vi "calculate virtual Z pos.vi"   [LabVIEW 2012]
uses:
  <vilib>/Analysis/coordinate.llb/Euler Rotation Order.ctl
  GFG/GFGnumericGet.vi
  <vilib>/Analysis/coordinate.llb/3D Cartesian Coordinate Rotation (Euler) (Scalar).vi
  <vilib>/Analysis/NI_AALPro.lvlib
  GFG/GFG library.lvlib
types:
  T1 = cluster{"Numeric":dbl, "Numeric":dbl, "Numeric":dbl}
  T2 = typedef "NI_AALPro.lvlib/Euler Rotation Order.ctl" = u16
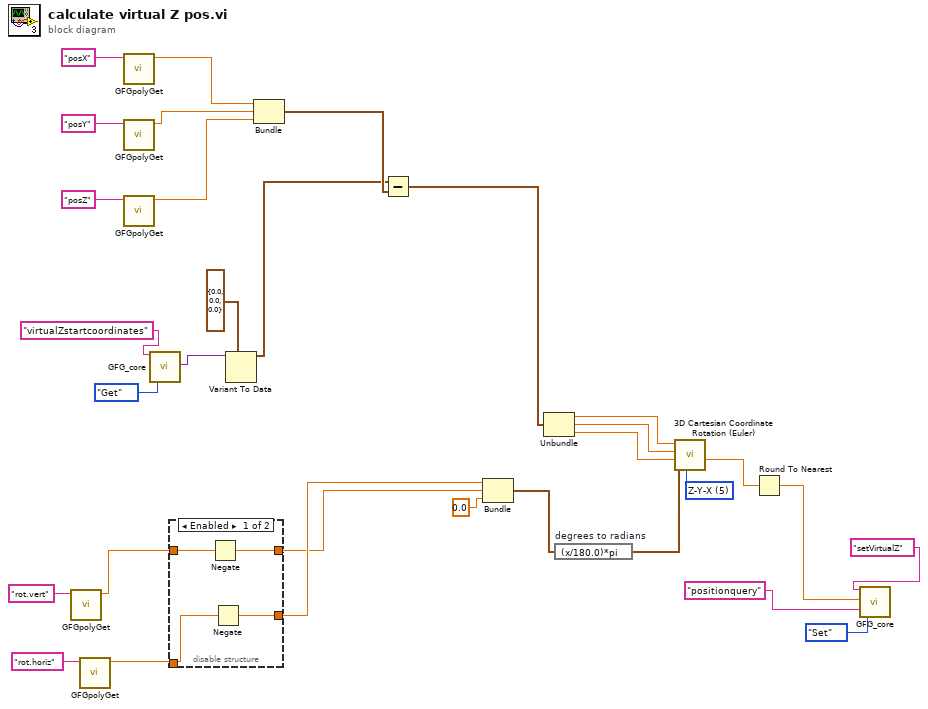
[diagram p0: block diagram]
diagram:
  w30 = T2 5 items=["X-Y-Z", "X-Z-Y", "Y-X-Z", "Y-Z-X", "Z-X-Y", "Z-Y-X", "X-Y-X", "X-Z-X", "Y-X-Y", "Y-Z-Y", "Z-X-Z", "Z-Y-Z"] ("rotation order")
  n1 = call-poly "GFGpolyGet.vi"("Variable Name in"="rot.vert") -> ("Numeric"=w14:dbl)  [unwired: 9 in, 1 out]
  n2 = call-poly "GFGpolyGet.vi"("Variable Name in"="rot.horiz") -> ("Numeric"=w15:dbl)  [unwired: 9 in, 1 out]
  n3 = call-poly "GFGpolyGet.vi"("Variable Name in"="posX") -> ("Numeric"=w22:dbl)  [unwired: 9 in, 1 out]
  n4 = call-poly "GFGpolyGet.vi"("Variable Name in"="posY") -> ("Numeric"=w21:dbl)  [unwired: 9 in, 1 out]
  n5 = call-poly "GFGpolyGet.vi"("Variable Name in"="posZ") -> ("Numeric"=w20:dbl)  [unwired: 9 in, 1 out]
  n6 = call "GFG_core.vi"("Variable Name in"="virtualZstartcoordinates", "Action"=enum16{"Init", "Set", "Get"}."Get") -> ("Variant Out"=w27:variant)  [unwired: 11 in, 6 out]
  n7 = disable-structure shown="Enabled" {
    disable-tunnel: w15 -> [w35 w36]
    disable-tunnel: w14 -> [w34 w37]
    disable-tunnel: [w33 w37] -> w7
    disable-tunnel: [w32 w36] -> w8
    frame Enabled {
      n8 = Negate(x=w34) -> (-x=w33:dbl)
      n9 = Negate(x=w35) -> (-x=w32:dbl)
    }
    frame Disabled {
    }
  }
  n10 = Variant To Data(type=T1 {"Numeric"=0.0, "Numeric"=0.0, "Numeric"=0.0} ("output cluster"), Variant=w27) -> (data=w18:T1)  [unwired: 1 in, 1 out]
  n11 = Bundle("Numeric"=w22, "Numeric"=w21, "Numeric"=w20) -> (w19:T1)  [unwired: 1 in]
  n12 = Subtract(x=w18, y=w19) -> (x-y=w13:T1)
  n13 = Bundle(w8, w7, "phi"=0.0) -> (w5:cluster{dbl, dbl, "phi":dbl})  [unwired: 1 in]
  n14 = Unbundle(w13) -> ("Numeric"=w12:dbl, "Numeric"=w11:dbl, "Numeric"=w10:dbl)
  n15 = expression code="(x/180.0)*pi" "degrees to radians"(w5) -> (w31:cluster{dbl, dbl, "phi":dbl})
  n16 = call-poly <vilib>:"3D Cartesian Coordinate Rotation (Euler).vi"("rotation order"=w30, "Euler Angles"=w31, "z"=w10, "y"=w11, "x"=w12) -> ("z out"=w9:dbl)  [unwired: 3 in, 3 out]
  n17 = Round To Nearest(number=w9) -> (nearest integer value=w1:dbl)
  n18 = call "GFG_core.vi"("Variable Name in"="setVirtualZ", "Variant in"=w1, "Source VI"="positionquery", "Action"=enum16{"Init", "Set", "Get"}."Set") -> ()  [unwired: 9 in, 7 out]
